vi "Pose3d_Exp_Orig.vi"(9 "Twist3d":T1, 11 "Pose3d":T2={"Translation3d"={"X"=0.0, "Y"=0.0, "Z"=0.0}, "Rotation3d"={"Q_quaternion"={"R"=1.0, "V"=[0.0, 0.0, 0.0]}}} {"Translation3d"."Z" format="%14.3f"; "Translation3d"."Y" format="%14.3f"; "Translation3d"."X" format="%14.3f"}) -> (3 "Updated Pose3d":T2={"Translation3d"={"X"=0.0, "Y"=0.0, "Z"=0.0}, "Rotation3d"={"Q_quaternion"={"R"=1.0, "V"=[0.0, 0.0, 0.0]}}} {"Translation3d"."Z" format="%14.3f"; "Translation3d"."Y" format="%14.3f"; "Translation3d"."X" format="%14.3f"})   [LabVIEW 2019]
doc: "Obtain a new Pose3d from a (constant curvature) velocity.\n\nThe twist is a change in pose in the robot's coordinate frame since the previous pose update. When the user runs exp() on the previous known field-relative pose with the argument being the twist, the user will receive the new field-relative pose.\n\n\"Exp\" represents the pose exponential, which is solving a differential equation moving the pose forward in time. Obtain a new Pose2d from a (constant curvature) velocity.\n\n\nPARAMETERS:\n--------------\n - POSE3D - current POSE data structure\n - TWIST 3D- TThe change in pose in the robot's coordinate frame since the previous pose update. For example, if a non-holonomic robot moves forward 0.01 meters and changes angle by 0.5 degrees since the previous pose update, the twist would be Twist3d(0.01, 0.0, 0.0, new new Rotation3d(0.0, 0.0, Units.degreesToRadians(0.5))).\n\nRETURNS:\n-----------\n- OUT POSE3D - The new pose of the robot."
uses:
  Trajectory_Library.lvlib
  <vilib>/Analysis/NI_AALBase.lvlib
  <vilib>/Analysis/Matrix/NI_Matrix.lvlib
  <vilib>/Analysis/Matrix/Numeric/Multiply/Multiply - RM,R.vi
  <vilib>/Analysis/Matrix/Numeric/Add/Add - RM,RM.vi
  <vilib>/Analysis/baseanly.llb/Real A x B.vi
  TypeDef/TRANSLATION3D.ctl
  TypeDef/QUATERNION.ctl
  TypeDef/ROTATION3D.ctl
  TypeDef/POSE3D.ctl
  TypeDef/TWIST3D.ctl
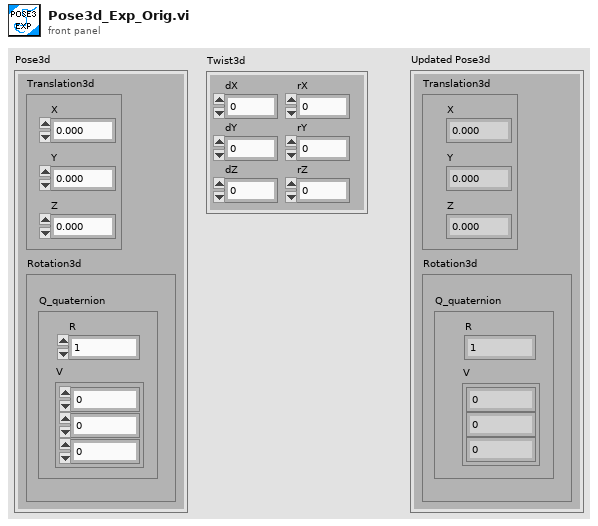
[diagram p1: front panel]
types:
  T1 = typedef "Trajectory_Library.lvlib/TWIST3D.ctl" = cluster{"dX":dbl, "dY":dbl, "dZ":dbl, "rX":dbl, "rY":dbl, "rZ":dbl}
  T2 = typedef "Trajectory_Library.lvlib/POSE3D.ctl" = cluster{"Translation3d":T3, "Rotation3d":T4}
  T3 = typedef "Trajectory_Library.lvlib/TRANSLATION3D.ctl" = cluster{"X":dbl, "Y":dbl, "Z":dbl}
  T4 = typedef "Trajectory_Library.lvlib/ROTATION3D.ctl" = cluster{"Q_quaternion":T5}
  T5 = typedef "Trajectory_Library.lvlib/QUATERNION.ctl" = cluster{"R":dbl, "V":dbl[]}
  T6 = typedef "NI_Matrix.lvlib/RealMatrix.ctl" = dbl[][]
  T7 = typedef "Trajectory_Library.lvlib/TRANSFORM3D.ctl" = cluster{"TRANSLATION3D":T3, "ROTATION3D":T4, "XF":bool}
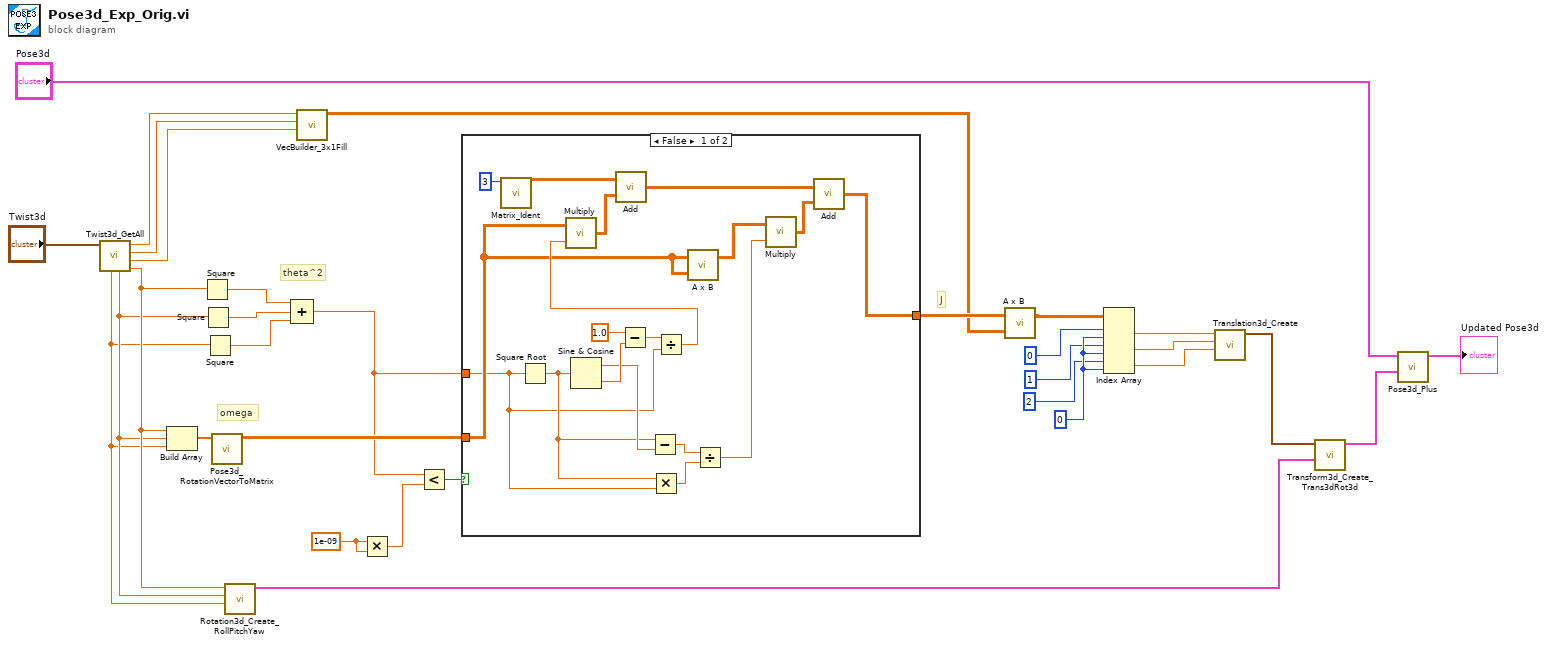
[diagram p0: block diagram]
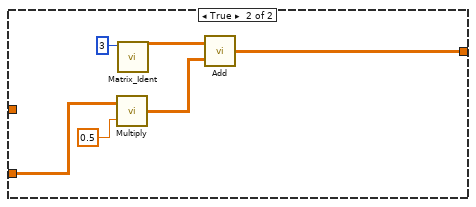
[diagram p2: hidden frame]
diagram:
  w9 = 0 ("index (col)")
  w25 = 1e-09 ("y")
  # "J"
  # "theta^2"
  # "omega"
  n1 = call "Twist3d_GetAll.vi"("Twist3d"="Twist3d") -> ("rX"=w3:dbl, "dZ"=w12:dbl, "dY"=w13:dbl, "dX"=w14:dbl, "rY"=w2:dbl, "rZ"=w1:dbl)  [unwired: 5 in]
  n2 = Build Array(w3, w2, w1) -> (w29:dbl[])
  n3 = Square(x=w3) -> (x^2=w28:dbl)
  n4 = Square(x=w2) -> (x^2=w27:dbl)
  n5 = Square(x=w1) -> (x^2=w26:dbl)
  n6 = call "Pose3d_RotationVectorToMatrix.vi"("RotationVector"=w29) -> ("Rotation Matrix"=w23:T6)  [unwired: 10 in]
  n7 = call "Rotation3d_Create_RollPitchYaw.vi"("Yaw"=w1, "Pitch"=w2, "Roll"=w3) -> ("Rotation3d"=w20:T4)  [unwired: 8 in]
  n8 = Compound Arithmetic op=ADD(w28, w27, w26) -> (w22:dbl)
  n9 = call "VecBuilder_3x1Fill.vi"("R2"=w12, "R1"=w13, "R0"=w14) -> ("output matrix"=w15:T6)  [unwired: 8 in]
  n10 = Multiply(x=w25, y=w25) -> (x*y=w24:dbl)
  n11 = Less?(x=w22, y=w24) -> (x < y?=w31:bool)
  n12 = case shown="False" w31 {
    tunnel: w23 -> [w39 w53]
    tunnel: [w32 w50] -> w16
    tunnel: w22 -> [w36 _]
    frame False {
      n13 = call "Matrix_Ident.vi"("Size"=3) -> ("output matrix"=w48:T6)  [unwired: 9 in, 1 out]
      n14 = Square Root(x=w36) -> (sqrt(x)=w37:dbl)
      n15 = Sine & Cosine(0:w37) -> (1:w38:dbl, 2:w46:dbl)
      n16 = Subtract(x=1.0, y=w46) -> (x-y=w45:dbl)
      n17 = Subtract(x=w37, y=w38) -> (x-y=w35:dbl)
      n18 = Multiply(x=w37, y=w36) -> (x*y=w34:dbl)
      n19 = Divide(x=w45, y=w36) -> (x/y=w43:dbl)
      n20 = call-poly <vilib>:"Multiply.vi"("Real Scalar c"=w43, "Real Matrix A"=w39) -> ("A * c"=w44:T6)
      n21 = call-poly <vilib>:"Add.vi"("Real Matrix B"=w44, "Real Matrix A"=w48) -> ("A + B"=w42:T6)
      n22 = call-poly <vilib>:"A x B.vi"("B"=w39, "A"=w39) -> ("A x B"=w41:T6)  [unwired: 1 out]
      n23 = Divide(x=w35, y=w34) -> (x/y=w33:dbl)
      n24 = call-poly <vilib>:"Multiply.vi"("Real Scalar c"=w33, "Real Matrix A"=w41) -> ("A * c"=w40:T6)
      n25 = call-poly <vilib>:"Add.vi"("Real Matrix B"=w40, "Real Matrix A"=w42) -> ("A + B"=w32:T6)
    }
    frame True {
      n26 = call-poly <vilib>:"Multiply.vi"("Real Scalar c"=0.5 ("y"), "Real Matrix A"=w53) -> ("A * c"=w51:T6)
      n27 = call "Matrix_Ident.vi"("Size"=3) -> ("output matrix"=w52:T6)  [unwired: 9 in, 1 out]
      n28 = call-poly <vilib>:"Add.vi"("Real Matrix B"=w51, "Real Matrix A"=w52) -> ("A + B"=w50:T6)
    }
  }
  n29 = call-poly <vilib>:"A x B.vi"("B"=w15, "A"=w16) -> ("A x B"=w11:T6)  [unwired: 1 out]
  n30 = Index Array(array=w11, index (row) #1=0 ("index (row)"), index (col) #1=w9, index (row) #2=1 ("index (row)"), index (col) #2=w9, index (row) #3=2 ("index (row)"), index (col) #3=w9) -> (element #1=w6:dbl, element #2=w5:dbl, element #3=w4:dbl)
  n31 = call "Translation3d_Create.vi"("Z"=w4, "Y"=w5, "X"=w6) -> ("TRANSLATION3D"=w21:T3)  [unwired: 8 in]
  n32 = call "Transform3d_Create_Trans3dRot3d.vi"("Rotation3d"=w20, "Translation3d"=w21) -> ("Transform3d"=w19:T7)  [unwired: 9 in]
  n33 = call "Pose3d_Plus.vi"("other Transform3d"=w19, "in Pose3d"="Pose3d") -> ("out Pose3d"=→"Updated Pose3d":T2)  [unwired: 9 in]
